vi "Validate IA Name Is Not In Use.vi"(8 "Error In":errorcluster, 10 "Name In":string, 11 "Instrument Addon Refnum In":T1 format="%.0x") -> (0 "Error Out":errorcluster, 2 "Name Out":string, 3 "Instrument Addon Refnum Out":T1=18446744073709551615 format="%.0x")   [LabVIEW 2018, in "Instrument Addon Scripting API.lvlib"]
doc: "Verifies if the desired name is already in use by a different Instrument Addon Custom Device.\n\nInput: \nInstrument Addon Refnum In: represents the reference to the Instrument Addon Custom Device\nName In: represents the desired name for the Custom Device\n\nOutput:\nInstrument Addon Refnum Our: represents the reference to the Instrument Addon Custom Device provided as input\nName Out: represents the desired name provided as input"
uses:
  Instrument Addon Scripting API.lvlib
  <vilib>/NI Veristand/Custom Device API/Custom Device Item Ref.ctl
  NationalInstruments.VeriStand.SystemDefinitionAPI
  Addon/Addon Shared/SubVIs/Constants.vi
  <vilib>/NI/NI VeriStand Advanced SysDef API/_SubVIs/SysDef.Search.GUIDs.vi
  <vilib>/Utility/error.llb/Error Cluster From Error Code.vi
  <vilib>/ErrorRing/Error Ring.xnode
  <vilib>/NI/NI VeriStand Advanced SysDef API/SysDef API/Advanced System Definition.lvlib
  Addon/Addon Shared/Instrument Addon Shared.lvlib
  <vilib>/NI Veristand/Custom Device API/Custom Device API.lvlib
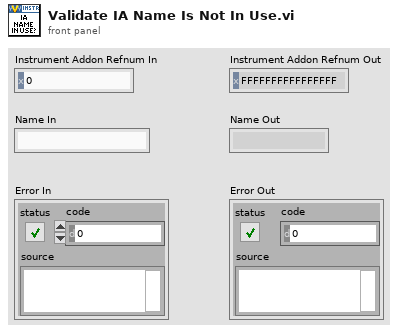
[diagram p1: front panel]
types:
  T1 = typedef "Custom Device API.lvlib/Custom Device Item Ref.ctl" = u64
  T2 = typedef "Advanced System Definition.lvlib/TreeItem.Info.ctl" = cluster{"Name":string, "Description":string, "GUID":string, "Is Channel":bool, "Channel":T3, "Is Waveform":bool, "Waveform":T5}
  T3 = typedef "Custom Device API.lvlib/Custom Device Channel.ctl" = cluster{"Type":T4, "Units":string, "Default Value":dbl, "Faultable":bool, "Scalable":bool}
  T4 = typedef "Custom Device API.lvlib/Custom Device Channel Type.ctl" = enum16{"Input", "Output"}
  T5 = typedef "Custom Device API.lvlib/Custom Device Waveform.ctl" = cluster{"Data Type":T6, "Units":string}
  T6 = typedef "Custom Device API.lvlib/Custom Device Waveform DataType.ctl" = enum16{"Double", "Complex Double"}
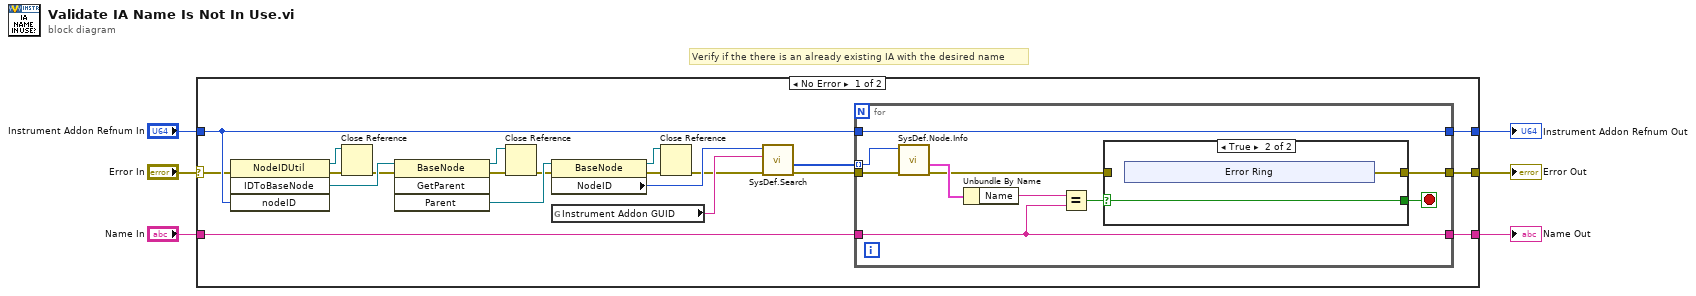
[diagram p0: block diagram]
diagram:
  # "Verify if the there is an already existing IA with the desired name"
  n1 = case shown="No Error" "Error In" {
    selector: "Error In" -> [w7 w48]
    tunnel: "Name In" -> [w23 w47]
    tunnel: [w20 w48] -> w5
    tunnel: [w19 w47] -> w4
    tunnel: "Instrument Addon Refnum In" -> [w18 w49]
    tunnel: [w17 w49] -> w2
    frame No Error {
      n2 = invoke class="NodeIDUtil" method="IDToBaseNode"(error in=w7, "nodeID"=w18) -> (reference out=w14:refnum<k24>, error out=w16:errorcluster, "IDToBaseNode"=w27:refnum<k24>)  [unwired: 2 in, 1 out]
      n3 = Close Reference(reference=w14, error in (no error)=w16) -> (error out=w15:errorcluster)
      n4 = invoke class="BaseNode" method="GetParent"(reference=w27, error in=w15) -> (reference out=w12:refnum<k24>, error out=w13:errorcluster, "Parent"=w26:refnum<k24>)  [unwired: 2 in, 1 out]
      n5 = Close Reference(reference=w12, error in (no error)=w13) -> (error out=w11:errorcluster)
      n6 = property class="BaseNode"(reference=w26, error in=w11) -> (reference out=w9:refnum<k24>, error out=w10:errorcluster, "NodeID"=w25:u64)
      n7 = global read "Constants.vi" "Instrument Addon GUID"() -> (w24:string)
      n8 = Close Reference(reference=w9, error in (no error)=w10) -> (error out=w8:errorcluster)
      n9 = call-poly <vilib>:"SysDef.Search.vi"("error in (no error)"=w8, "GUID"=w24, "nodeID"=w25) -> ("error out"=w22:errorcluster, "Values Out"=w21:u64[])  [unwired: 5 in, 2 out]
      n10 = for {
        tunnel: w23 -> [w29]
        tunnel: w22 -> [w37]
        tunnel: w21 -> [w36] mode=indexing
        tunnel: [w30] -> w20
        tunnel: [w29] -> w19
        tunnel: w18 -> [w28]
        tunnel: [w28] -> w17
        stop <- w31 stop-if-true
        n11 = call <vilib>:"SysDef.Node.Info.vi"("error in (no error)"=w37, "nodeID"=w36) -> ("error out"=w32:errorcluster, "Item Info"=w35:T2)  [unwired: 6 in, 2 out]
        n12 = Unbundle By Name(w35) -> ("Name"=w34:string)
        n13 = Equal?(x=w34, y=w29) -> (x = y?=w33:bool)
        n14 = case shown="True" w33 {
          selector: w33 -> [w38 w41]
          tunnel: w32 -> [w39 _]
          tunnel: [w38 w41] -> w31
          tunnel: [w39 w40] -> w30
          frame False {
          }
          frame True {
            n15 = xnode "Error Ring"() -> ("error out"=w40:errorcluster)
          }
        }
      }
    }
    frame Error {
    }
  }
  "Error Out" <- w5
  "Name Out" <- w4
  "Instrument Addon Refnum Out" <- w2
